vi "Check for Environment Errors.vi"(8 "error in (no error)":errorcluster) -> (0 "error out":errorcluster)   [LabVIEW 2020, in "jki_python_bridge.lvlib" / "Server.lvclass"]
uses:
  Server.lvclass
  Server.lvclass/Server.ctl
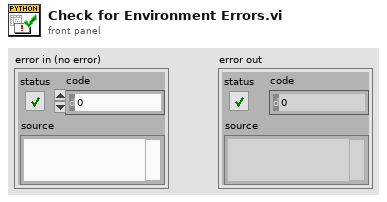
[diagram p1: front panel]
types:
  T1 = enum32{"invalid app kind", "Development System", "Run Time System", "Student Edition", "Embedded LabVIEW", "Evaluation", "Custom"}
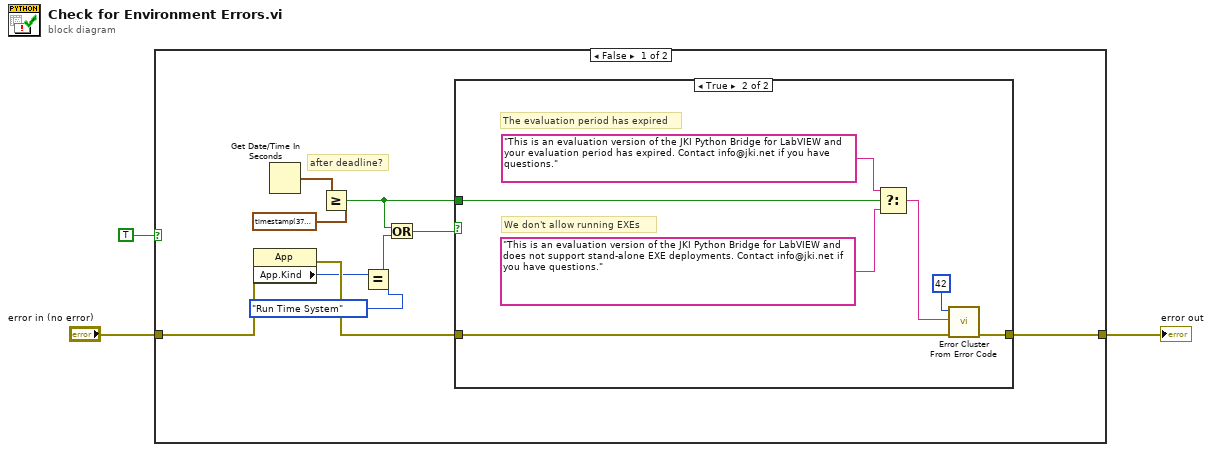
[diagram p0: block diagram]
diagram:
  n1 = case shown="False" TRUE {
    tunnel: [w4 w22] -> w3
    tunnel: "error in (no error)" -> [w5 w22]
    frame False {
      # "after deadline?"
      n2 = property class="App"(error in=w5) -> (error out=w11:errorcluster, "App.Kind"=w8:T1)  [unwired: 1 in, 1 out]
      n3 = Get Date/Time In Seconds() -> (seconds since 1Jan1904=w9:timestamp)
      n4 = Greater Or Equal?(x=w9, y=timestamp(3707971200 s since 1904-01-01) ("current time")) -> (x >= y?=w13:bool)
      n5 = Equal?(x=w8, y=T1."Run Time System" ("App.Kind")) -> (x = y?=w12:bool)
      n6 = Or(x=w13, y=w12) -> (x .or. y?=w10:bool)
      n7 = case shown="True" w10 {
        tunnel: w11 -> [w14 w20]
        tunnel: [w14 w19] -> w4
        tunnel: w13 -> [_ w15]
        frame False {
        }
        frame True {
          # "We don't allow running EXEs"
          # "The evaluation period has expired"
          n8 = Select(t="This is an evaluation version of the JKI Python Bridge for LabVIEW and your evaluation period has expired. Contact info@jki.net if you have questions." ("String to Prepend to source (\"\")"), s=w15, f="This is an evaluation version of the JKI Python Bridge for LabVIEW and does not support stand-alone EXE deployments. Contact info@jki.net if you have questions." ("String to Prepend to source (\"\")")) -> (s? t:f=w16:string)
          n9 = call <vilib>:"Error Cluster From Error Code.vi"("error in (no error)"=w20, "error message (\"\")"=w16, "error code (0)"=42 ("code")) -> ("error out"=w19:errorcluster)  [unwired: 6 in]
        }
      }
    }
    frame True {
    }
  }
  "error out" <- w3
